vi "Tosca-Launcher.vi"() -> ()   [LabVIEW 2020]
uses:
  <resource>/objmgr/daqmx.rc
panel:
  out "Loading":string
  out "Version":string
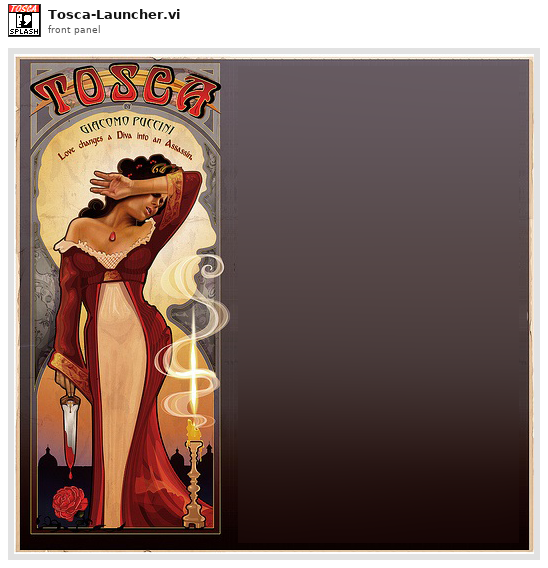
[diagram p1: front panel]
types:
  T1 = cluster{"Major":i32, "Minor":i32, "Build":i32, "Private":i32, "FileVersion":string, "ProductName":string, "InternalName":string, "CompanyName":string, "LegalCopyright":string, "FileDescription":string}
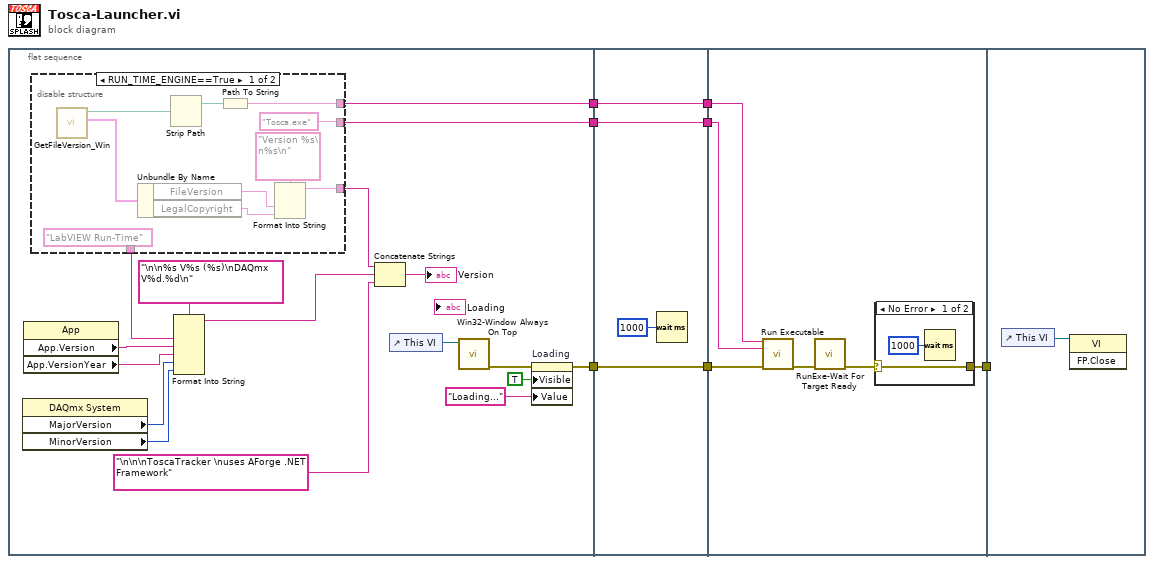
[diagram p0: block diagram]
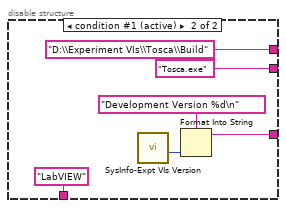
[diagram p2: hidden frame]
diagram:
  n1 = flat-sequence {
    tunnel: [w22] -> w6
    tunnel: [w20] -> w4
    tunnel: [w19] -> w2
    tunnel: [w44] -> w7
    tunnel: w6 -> [w44]
    tunnel: [w43] -> w5
    tunnel: w4 -> [w43]
    tunnel: [w42] -> w3
    tunnel: w2 -> [w42]
    tunnel: w7 -> [w48]
    tunnel: w5 -> [w47]
    tunnel: w3 -> [w46]
    tunnel: [w45] -> w1
    tunnel: w1 -> [_]
    frame #0 {
      n2 = property class="DAQmx System"() -> ("MajorVersion"=w17:u32, "MinorVersion"=w18:u32)  [unwired: 2 in, 2 out]
      n3 = property class="App"() -> ("App.Version"=w15:string, "App.VersionYear"=w16:string)  [unwired: 2 in, 2 out]
      n4 = disable-structure shown="RUN_TIME_ENGINE==True" {
        disable-tunnel: [w32 w38] -> w13
        disable-tunnel: ["LabVIEW Run-Time" "LabVIEW"] -> w10
        disable-tunnel: [w25 "D:\\Experiment VIs\\Tosca\\Build" ("Folder")] -> w20
        disable-tunnel: ["Tosca.exe" (".EXE name") "Tosca.exe" (".EXE name")] -> w19
        frame condition #0 {
          n5 = call "GetFileVersion_Win.vi"() -> ("File Info Out"=w33:T1, "Exe Path Out"=w28:path)  [unwired: 9 in, 1 out]
          n6 = Unbundle By Name(w33) -> ("FileVersion"=w31:string, "LegalCopyright"=w30:string)
          n7 = Strip Path(path=w28) -> (stripped path=w26:path)  [unwired: 1 out]
          n8 = Path To String(path=w26) -> (string=w25:string)
          n9 = Format Into String(format string="Version %s\n%s\n", w31, w30) -> (resulting string=w32:string)  [unwired: 2 in, 1 out]
        }
        frame condition #1 (active) {
          n10 = call "SysInfo-Expt VIs Version.vi"() -> ("Expt VIs Version out"=w39:i32)  [unwired: 11 in]
          n11 = Format Into String(format string="Development Version %d\n" ("PF Version"), w39) -> (resulting string=w38:string)  [unwired: 2 in, 1 out]
        }
      }
      n12 = Format Into String(format string="\n\n%s V%s (%s)\nDAQmx V%d.%d\n", w10, w15, w16, w17, w18) -> (resulting string=w12:string)  [unwired: 2 in, 1 out]
      n13 = Concatenate Strings(w13, w12, "\n\n\nToscaTracker \nuses AForge .NET Framework" ("string")) -> (→"Version":string)
      n14 = control-ref of="This VI"() -> (w9:refnum<vi>)
      n15 = call "Win32-Window Always On Top.vi"("VI reference"=w9) -> ("error out"=w21:errorcluster)  [unwired: 10 in]
      n16 = property on="Loading" class="Str"(error in=w21, "Visible"=TRUE, "Value"="Loading..." ("Loading")) -> (error out=w22:errorcluster)  [unwired: 1 in, 1 out]
    }
    frame #1 {
      n17 = Wait (ms)(milliseconds to wait=u32 1000) -> ()  [unwired: 1 out]
    }
    frame #2 {
      n18 = call "Run Executable.vi"("Folder"=w47, ".EXE name"=w46, "error in (no error)"=w48) -> ("error out"=w49:errorcluster)  [unwired: 12 in]
      n19 = call "RunExe-Wait For Target Ready.vi"("error in (no error)"=w49) -> ("error out"=w50:errorcluster)  [unwired: 14 in]
      n20 = case shown="No Error" w50 {
        selector: w50 -> [w51 w53]
        tunnel: [w51 w53] -> w45
        frame No Error {
          n21 = Wait (ms)(milliseconds to wait=u32 1000) -> ()  [unwired: 1 out]
        }
        frame Error {
        }
      }
    }
    frame #3 {
      n22 = control-ref of="This VI"() -> (w54:refnum<vi>)
      n23 = invoke class="VI" method="FP.Close"(reference=w54) -> ()  [unwired: 2 in, 3 out]
    }
  }
